vi "Normalize Scheme Port.vi"(11 "URI In":refnum<class "URI.lvclass">) -> (3 "URI":refnum<class "URI.lvclass">)   [LabVIEW 2020, in "HTTP Utils.lvlib"]
uses:
  HTTP Utils.lvlib
  lv-stream/stream/URI/URI.lvclass
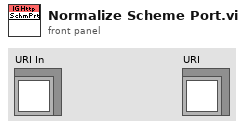
[diagram p1: front panel]
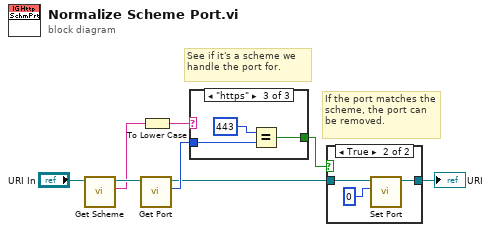
[diagram p0: block diagram]
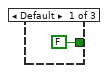
[diagram p3: hidden frame]
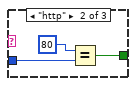
[diagram p4: hidden frame]
diagram:
  # "If the port matches the scheme, the port can be removed."
  # "See if it's a scheme we handle the port for."
  n1 = call "Get Scheme.vi"("URI in"="URI In") -> ("Scheme"=w6:string, "URI out"=w7:refnum<class "URI.lvclass">)  [unwired: 8 in, 1 out]
  n2 = call "Get Port.vi"("URI in"=w7) -> ("Port"=w4:u16, "URI out"=w3:refnum<class "URI.lvclass">)  [unwired: 8 in, 1 out]
  n3 = To Lower Case(string=w6) -> (all lower case string=w5:string)
  n4 = case shown="\"https\"" w5 {
    tunnel: w4 -> [_ w12 w15]
    tunnel: [FALSE w10 w13] -> w2
    frame Default {
    }
    frame "http" {
      n5 = Equal?(x=u16 80 ("y"), y=w12) -> (x = y?=w10:bool)
    }
    frame "https" {
      n6 = Equal?(x=u16 443 ("y"), y=w15) -> (x = y?=w13:bool)
    }
  }
  n7 = case shown="True" w2 {
    tunnel: w3 -> [w16 w19]
    tunnel: [w16 w17] -> w1
    frame False {
    }
    frame True {
      n8 = call "Set Port.vi"("Port"=u16 0, "URI in"=w19) -> ("URI out"=w17:refnum<class "URI.lvclass">)  [unwired: 8 in, 1 out]
    }
  }
  "URI" <- w1
